vi "performance data.vi"(11 "CPU %":sgl) -> (0 "Dash IPS":u32, 1 "Dash mSPI":u32, 2 "Main IPS":u32, 3 "Main mSPI":u32, 5 "Stats":sgl[][](graph))   [LabVIEW 2015]
uses:
  <vilib>/Rock Robotics/Network Tables/NT Read Numeric Array.vi
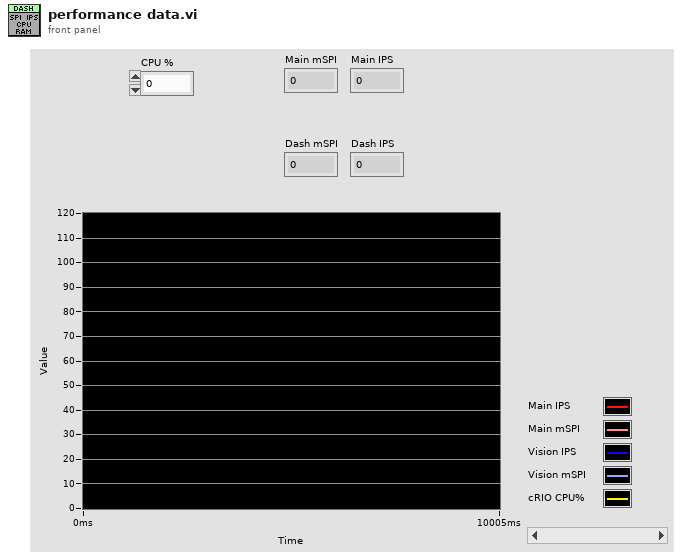
[diagram p1: front panel]
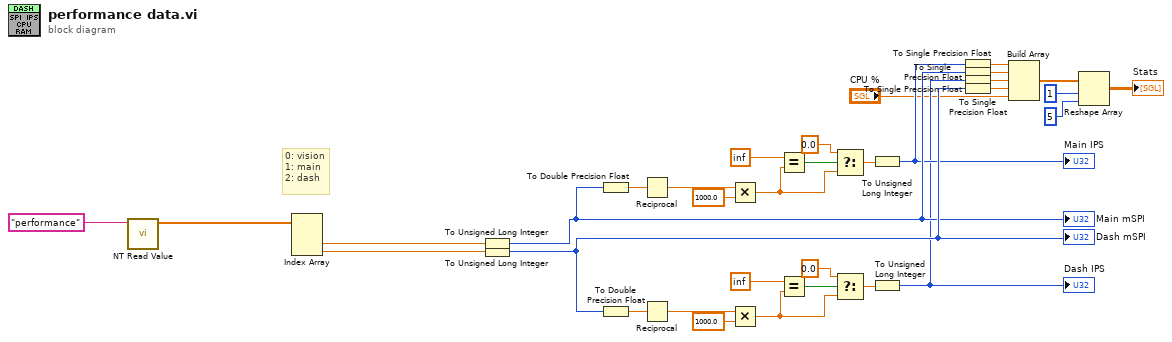
[diagram p0: block diagram]
diagram:
  # "0: vision\n1: main\n2: dash"
  n1 = call-poly <vilib>:"NT Read Value.vi"("Name"="performance") -> ("Numeric Array"=w11:dbl[])  [unwired: 9 in, 1 out]
  n2 = Index Array(array=w11) -> (element #2=w9:dbl, element #3=w10:dbl)  [unwired: 3 in, 1 out]
  n3 = To Unsigned Long Integer(number=w9) -> (unsigned 32bit integer=w32:u32)
  "Main mSPI" <- w32
  n4 = To Unsigned Long Integer(number=w10) -> (unsigned 32bit integer=w33:u32)
  "Dash mSPI" <- w33
  n5 = To Double Precision Float(number=w32) -> (double precision float=w29:dbl)
  n6 = To Double Precision Float(number=w33) -> (double precision float=w22:dbl)
  n7 = Reciprocal(x=w29) -> (1/x=w30:dbl)
  n8 = Reciprocal(x=w22) -> (1/x=w21:dbl)
  n9 = Multiply(x=w30, y=1000.0) -> (x*y=w14:dbl)
  n10 = Multiply(x=w21, y=1000.0) -> (x*y=w13:dbl)
  n11 = Equal?(x=inf, y=w14) -> (x = y?=w28:bool)
  n12 = Equal?(x=inf, y=w13) -> (x = y?=w23:bool)
  n13 = Select(t=0.0, s=w28, f=w14) -> (s? t:f=w19:dbl)
  n14 = Select(t=0.0, s=w23, f=w13) -> (s? t:f=w18:dbl)
  n15 = To Unsigned Long Integer(number=w19) -> (unsigned 32bit integer=w17:u32)
  "Main IPS" <- w17
  n16 = To Unsigned Long Integer(number=w18) -> (unsigned 32bit integer=w16:u32)
  "Dash IPS" <- w16
  n17 = To Single Precision Float(number=w17) -> (single precision float=w1:sgl)
  n18 = To Single Precision Float(number=w32) -> (single precision float=w2:sgl)
  n19 = To Single Precision Float(number=w16) -> (single precision float=w3:sgl)
  n20 = To Single Precision Float(number=w33) -> (single precision float=w4:sgl)
  n21 = Build Array(w1, w2, w3, w4, "CPU %") -> (w6:sgl[])
  n22 = Reshape Array(w6, 1 ("dimension size"), 5 ("dimension size")) -> (→"Stats":sgl[][])
